vi "rot1dArray.vi"(8 "error in (no error)":errorcluster, 9 "Rot Mat":dbl[][](array[numeric]), 10 "1D Array":dbl[](array[numeric]), 11 "MatOper in":refnum<class "MatOper.lvclass">) -> (0 "error out":errorcluster, 2 "Rotated 1D Array":dbl[](array[numeric]), 3 "MatOper out":refnum<class "MatOper.lvclass">)   [LabVIEW 2016, in "MatOper.lvclass"]
doc: "Rotate the 1D array based on the rotation matrix."
uses:
  MatOper.lvclass
  <vilib>/Analysis/baseanly.llb/Real A x B.vi
  <vilib>/Analysis/Matrix/Numeric/Conversions/Array To Matrix - RA2.vi
  <vilib>/Analysis/Matrix/Numeric/Conversions/Matrix To Array - RM.vi
  <vilib>/Analysis/Matrix/NI_Matrix.lvlib
  <vilib>/Analysis/NI_AALBase.lvlib
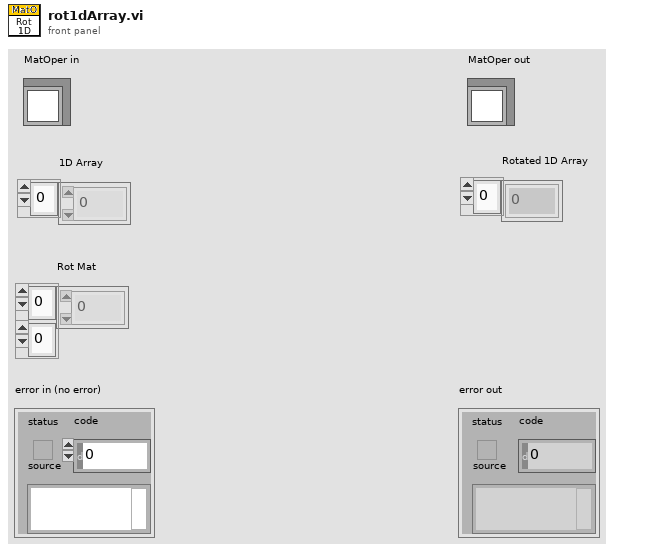
[diagram p1: front panel]
types:
  T1 = typedef "NI_Matrix.lvlib/RealMatrix.ctl" = dbl[][]
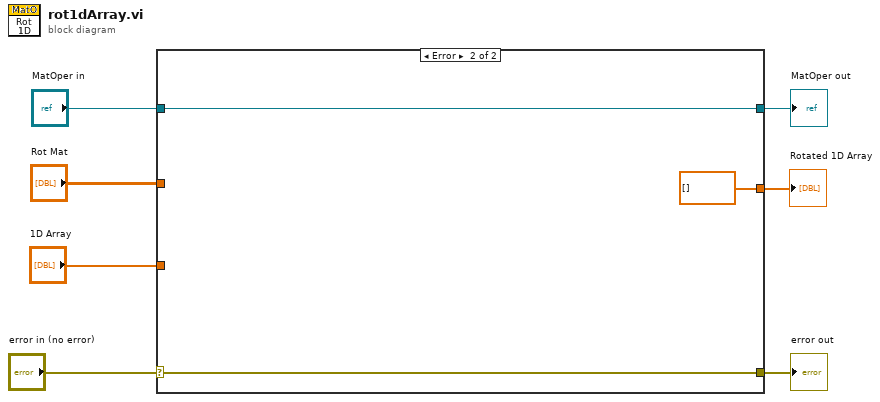
[diagram p0: block diagram]
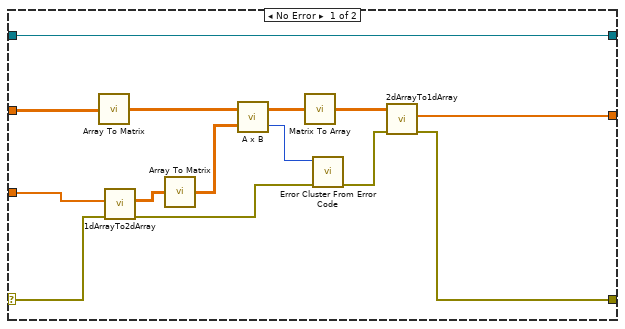
[diagram p2: hidden frame]
diagram:
  n1 = case shown="Error" "error in (no error)" {
    selector: "error in (no error)" -> [w11 w24]
    tunnel: [w8 w24] -> w6
    tunnel: [w21 w23] -> w4
    tunnel: "MatOper in" -> [w21 w23]
    tunnel: [w14 dbl[] [] ("1D Array")] -> w3
    tunnel: "1D Array" -> [w13 _]
    tunnel: "Rot Mat" -> [w12 _]
    frame No Error {
      n2 = call-poly <vilib>:"Array To Matrix.vi"("Real 2D Array"=w12) -> ("Real Matrix"=w19:T1)
      n3 = call "1dArrayTo2dArray.vi"("error in (no error)"=w11, "1D Array"=w13) -> ("error out"=w10:errorcluster, "2D Array"=w20:dbl[][])  [unwired: 7 in, 1 out]
      n4 = call-poly <vilib>:"Array To Matrix.vi"("Real 2D Array"=w20) -> ("Real Matrix"=w18:T1)
      n5 = call-poly <vilib>:"A x B.vi"("B"=w18, "A"=w19) -> ("error"=w17:i32, "A x B"=w16:T1)
      n6 = call-poly <vilib>:"Matrix To Array.vi"("Real Matrix"=w16) -> ("Real 2D Array"=w15:dbl[][])
      n7 = call <vilib>:"Error Cluster From Error Code.vi"("error in (no error)"=w10, "error code (0)"=w17) -> ("error out"=w9:errorcluster)  [unwired: 7 in]
      n8 = call "2dArrayTo1dArray.vi"("error in (no error)"=w9, "2D Array"=w15) -> ("error out"=w8:errorcluster, "1D Array"=w14:dbl[])  [unwired: 7 in, 1 out]
    }
    frame Error {
    }
  }
  "error out" <- w6
  "MatOper out" <- w4
  "Rotated 1D Array" <- w3
